vi "nanocal -- nuclear schottky fit V7.vi"() -> ()   [LabVIEW 2021] (continued)
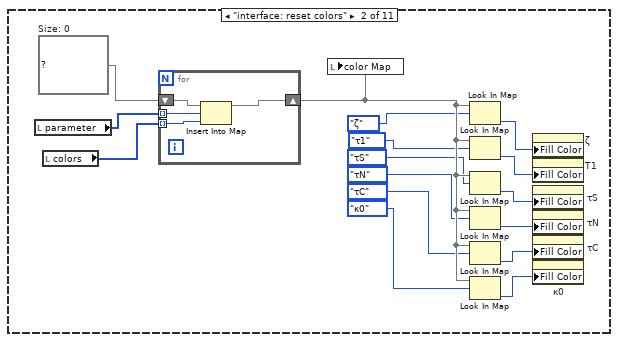
[diagram p3: hidden frame]
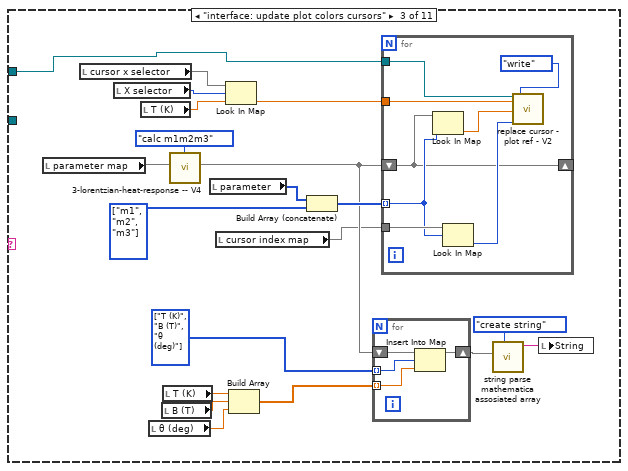
[diagram p4: hidden frame]
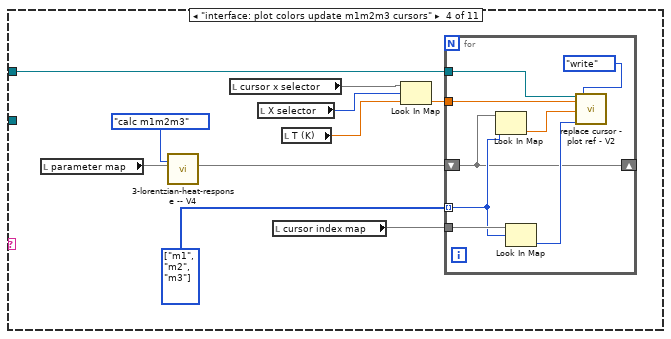
[diagram p5: hidden frame]
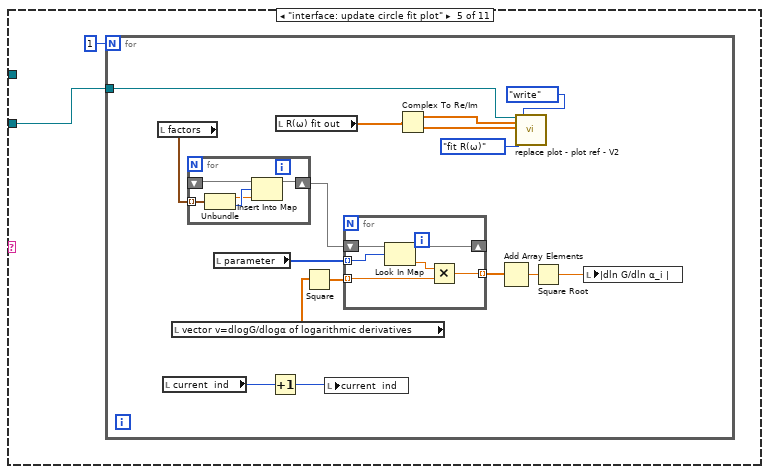
[diagram p6: hidden frame]
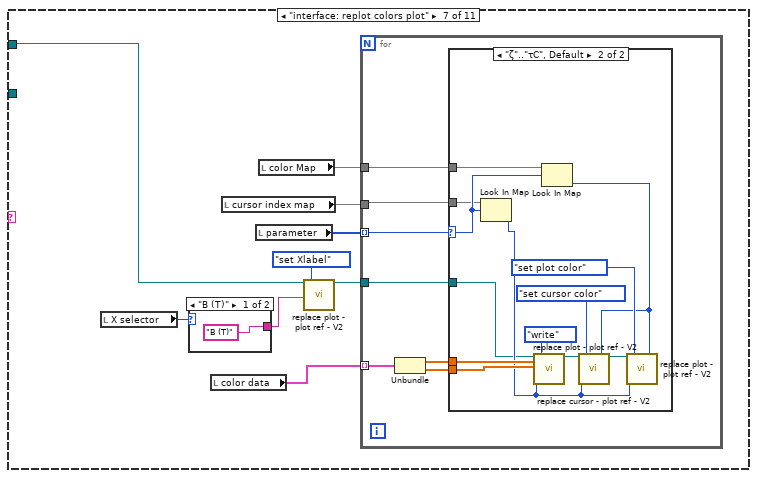
[diagram p8: hidden frame]
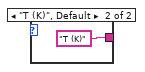
[diagram p9: hidden frame]
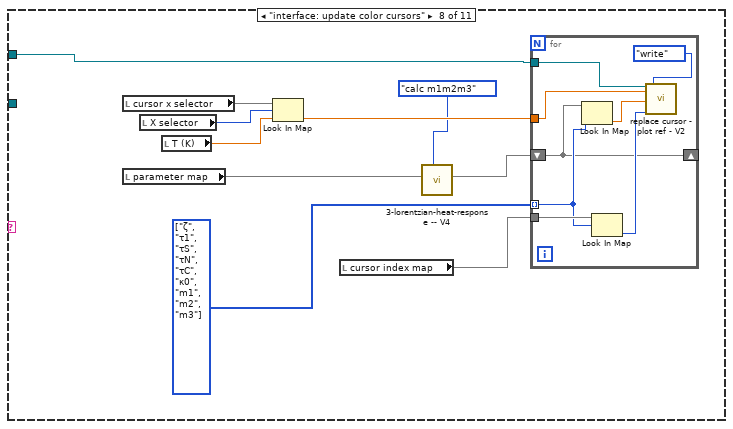
[diagram p11: hidden frame]
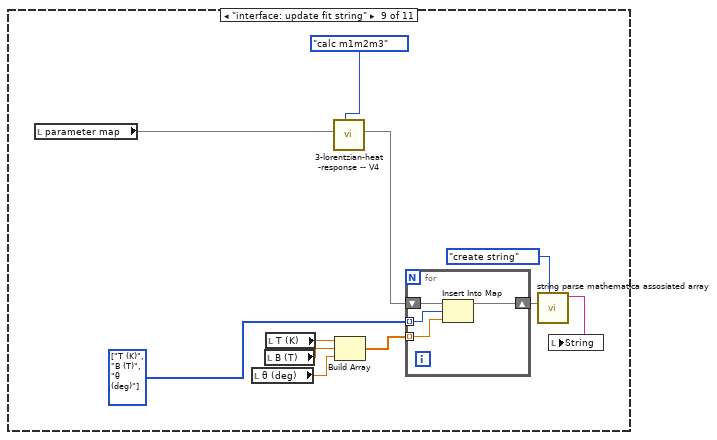
[diagram p12: hidden frame]
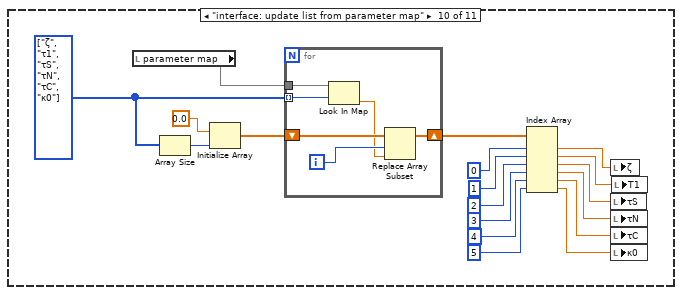
[diagram p13: hidden frame]
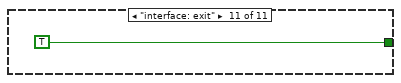
[diagram p14: hidden frame]
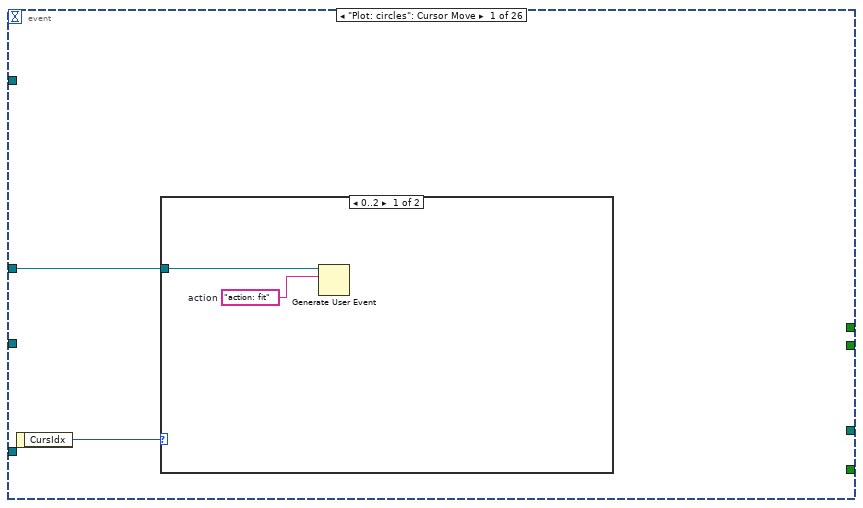
[diagram p15: hidden frame]
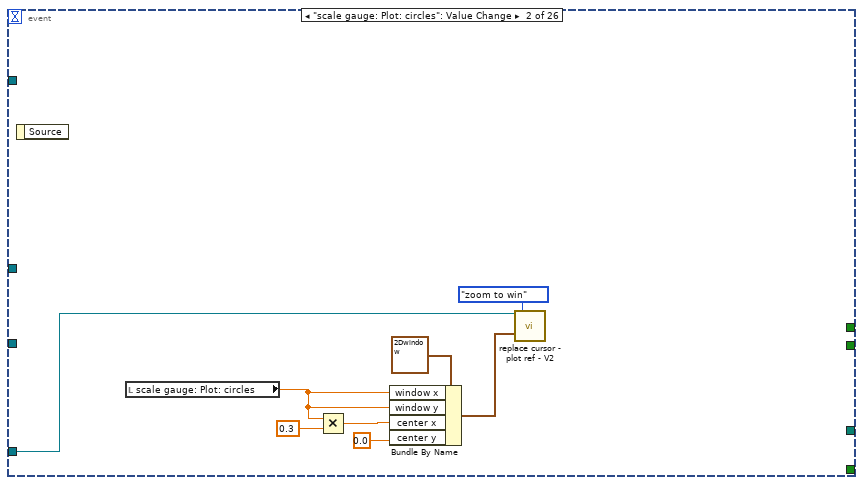
[diagram p17: hidden frame]
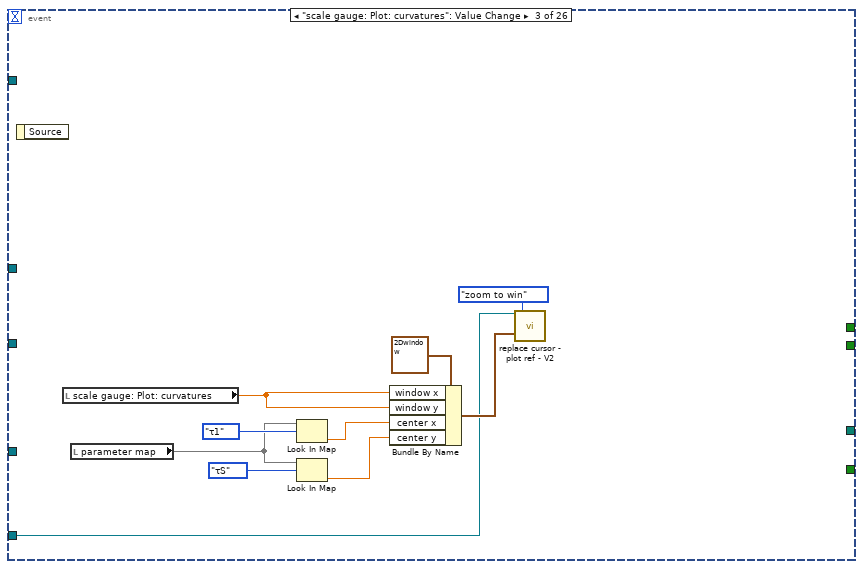
[diagram p18: hidden frame]
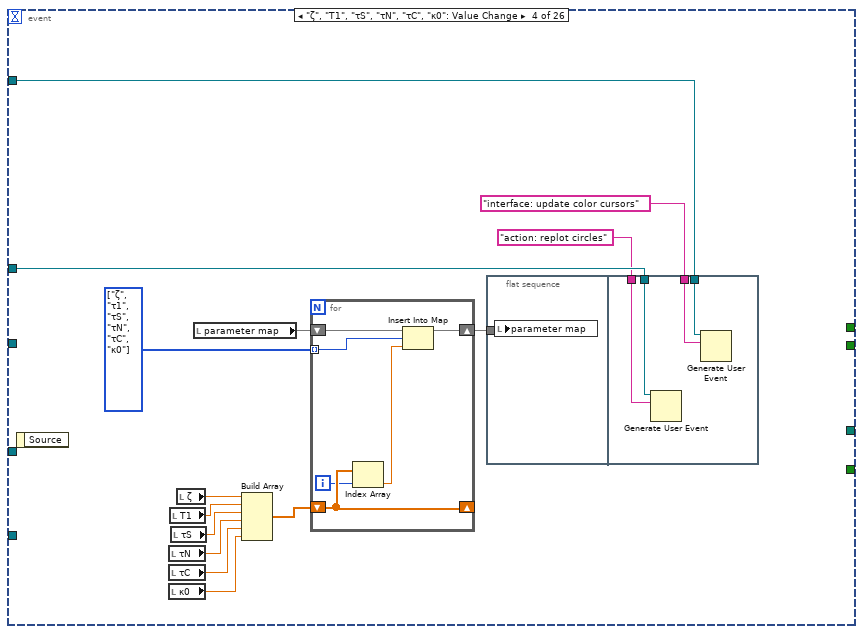
[diagram p19: hidden frame]
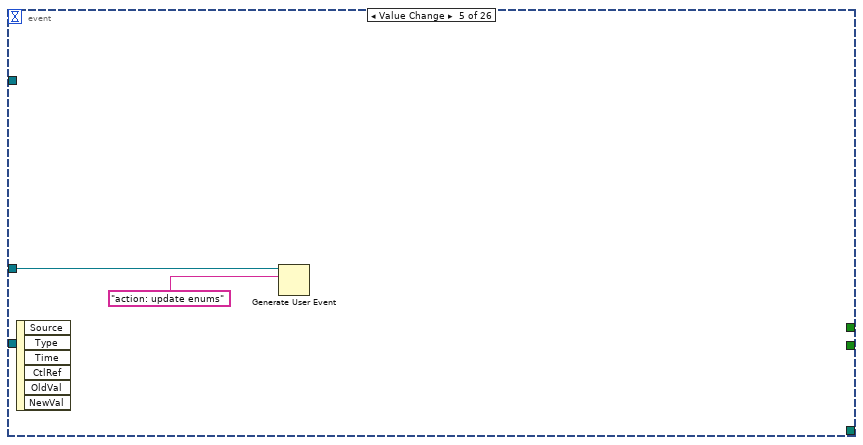
[diagram p20: hidden frame]
      event "Plot:  colors": Cursor Release {
        n776 = event-data() -> ("CursIdx"=w1534:i32)  [unwired: 1 in]
        n777 = local read "reverse cursor index map"() -> (w1535:map{i32, T2})
        n778 = call "replace cursor - plot ref - V2.vi"("Plot ref in"=w1536, "cursor index"=w1534, "cursor action"=cursor_action."read") -> ("read Y"=w1533:dbl)  [unwired: 13 in, 3 out]
        n779 = local read "parameter map"() -> (w1532:map{T2, dbl})
        n780 = Look In Map(map=w1535, key=w1534) -> (value=w1530:T2)  [unwired: 1 in, 1 out]
        n781 = in-place {
          in-place-border: w1533 -> [w1546]
          in-place-border: LVMapReplaceAction."Modify Entry only if found" ("action") -> [w1545]
          n782 = in-place-map #10(w1532, w1530) -> ()  [unwired: 1 in, 2 out]
          n783 = in-place-map #10(w1546, w1545) -> (w1531:map{T2, dbl})  [unwired: 2 out]
        }
        n784 = flat-sequence {
          tunnel: w1531 -> [w1538]
          tunnel: w1528 -> [w1544]
          tunnel: "action: replot circles" ("event data") -> [w1543]
          tunnel: w1526 -> [w1542]
          tunnel: "interface: update list from parameter map" ("event data") -> [w1541]
          tunnel: "interface: plot colors update m1m2m3 cursors" ("event data") -> [w1539]
          frame #0 {
            n785 = local write "parameter map"(w1538) -> ()
          }
          frame #1 {
            n786 = Generate User Event(user event=w1544, event data cluster=w1543) -> ()  [unwired: 2 in, 2 out]
            n787 = Generate User Event(user event=w1542, event data cluster=w1541) -> (user event out=w1540:refnum<user-event>)  [unwired: 2 in, 1 out]
            n788 = Generate User Event(user event=w1540, event data cluster=w1539) -> ()  [unwired: 2 in, 2 out]
          }
        }
      }
      event "Math→τ! :q": Value Change {
        n789 = event-data() -> ()  [unwired: 1 in, 1 out]
        n790 = Generate User Event(user event=w1548, event data cluster="action: copy from math" ("event data")) -> ()  [unwired: 2 in, 2 out]
      }
      event "load default values": Value Change {
        n791 = event-data() -> ()  [unwired: 1 in, 1 out]
        n792 = Generate User Event(user event=w1550, event data cluster="action: update default values" ("event data")) -> ()  [unwired: 2 in, 2 out]
      }
      event "τ→Math! :p": Value Change {
        n793 = event-data() -> ()  [unwired: 1 in, 1 out]
        n794 = Generate User Event(user event=w1554, event data cluster="action: copy to math" ("event data")) -> ()  [unwired: 2 in, 2 out]
      }
      event "Math→ string OUT! :s": Value Change {
        n795 = event-data() -> ()  [unwired: 1 in, 1 out]
        n796 = Generate User Event(user event=w1557, event data cluster="action: write mathematica string" ("event data")) -> ()  [unwired: 2 in, 2 out]
      }
      event "generate empty string from filelist !": Value Change {
        n797 = event-data() -> ()  [unwired: 1 in, 1 out]
        n798 = Generate User Event(user event=w1560, event data cluster="action: empty string from filelist" ("event data")) -> ()  [unwired: 2 in, 2 out]
      }
      event "string IN → Math!": Value Change {
        n799 = event-data() -> ()  [unwired: 1 in, 1 out]
        n800 = Generate User Event(user event=w1563, event data cluster="action: read mathematica string" ("event data")) -> ()  [unwired: 2 in, 2 out]
      }
      event "filenames": Value Change {
        n801 = event-data() -> ()  [unwired: 1 in, 1 out]
        n802 = local read "filesnames lookup"() -> (w1570:map{i32, string})
        n803 = local read "all full filenames"() -> (w1568:map{string, path})
        n804 = local read "filenames"() -> (w1569:u16)
        n805 = Look In Map(map=w1570, key=w1569) -> (value=w1567:string)  [unwired: 1 in, 1 out]
        n806 = Look In Map(map=w1568, key=w1567) -> (value=w1565:path)  [unwired: 1 in, 1 out]
        n807 = for {
          N: 1 -> [_]
          tunnel: w1571 -> [w1573]
          tunnel: w1565 -> [w1572]
          n808 = local write "Read from file"(w1572) -> ()
          n809 = Generate User Event(user event=w1573, event data cluster="action: read from file" ("event data")) -> ()  [unwired: 2 in, 2 out]
        }
      }
      event "selection :|\\": Value Change {
        n810 = event-data() -> ()  [unwired: 1 in, 1 out]
        n811 = Generate User Event(user event=w1575, event data cluster="action: constrained filenames select" ("event data")) -> ()  [unwired: 2 in, 2 out]
      }
      event "plot landscape!", "range one", "range two": Value Change {
        n812 = event-data() -> ()  [unwired: 1 in, 6 out]
        n813 = Generate User Event(user event=w1577, event data cluster="action: plot landscape" ("event data")) -> ()  [unwired: 2 in, 2 out]
      }
      event "colors": Value Change {
        n814 = event-data() -> ()  [unwired: 1 in, 6 out]
        n815 = Generate User Event(user event=w1580, event data cluster="action: reset colors" ("event data")) -> ()  [unwired: 2 in, 2 out]
      }
    }
  }
  "cursor x selector" <- w36
